vi "refocusProgram.vi"(8 "error in (no error)":errorcluster) -> ()   [LabVIEW 2022 SP3]
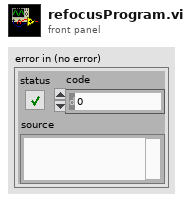
[diagram p1: front panel]
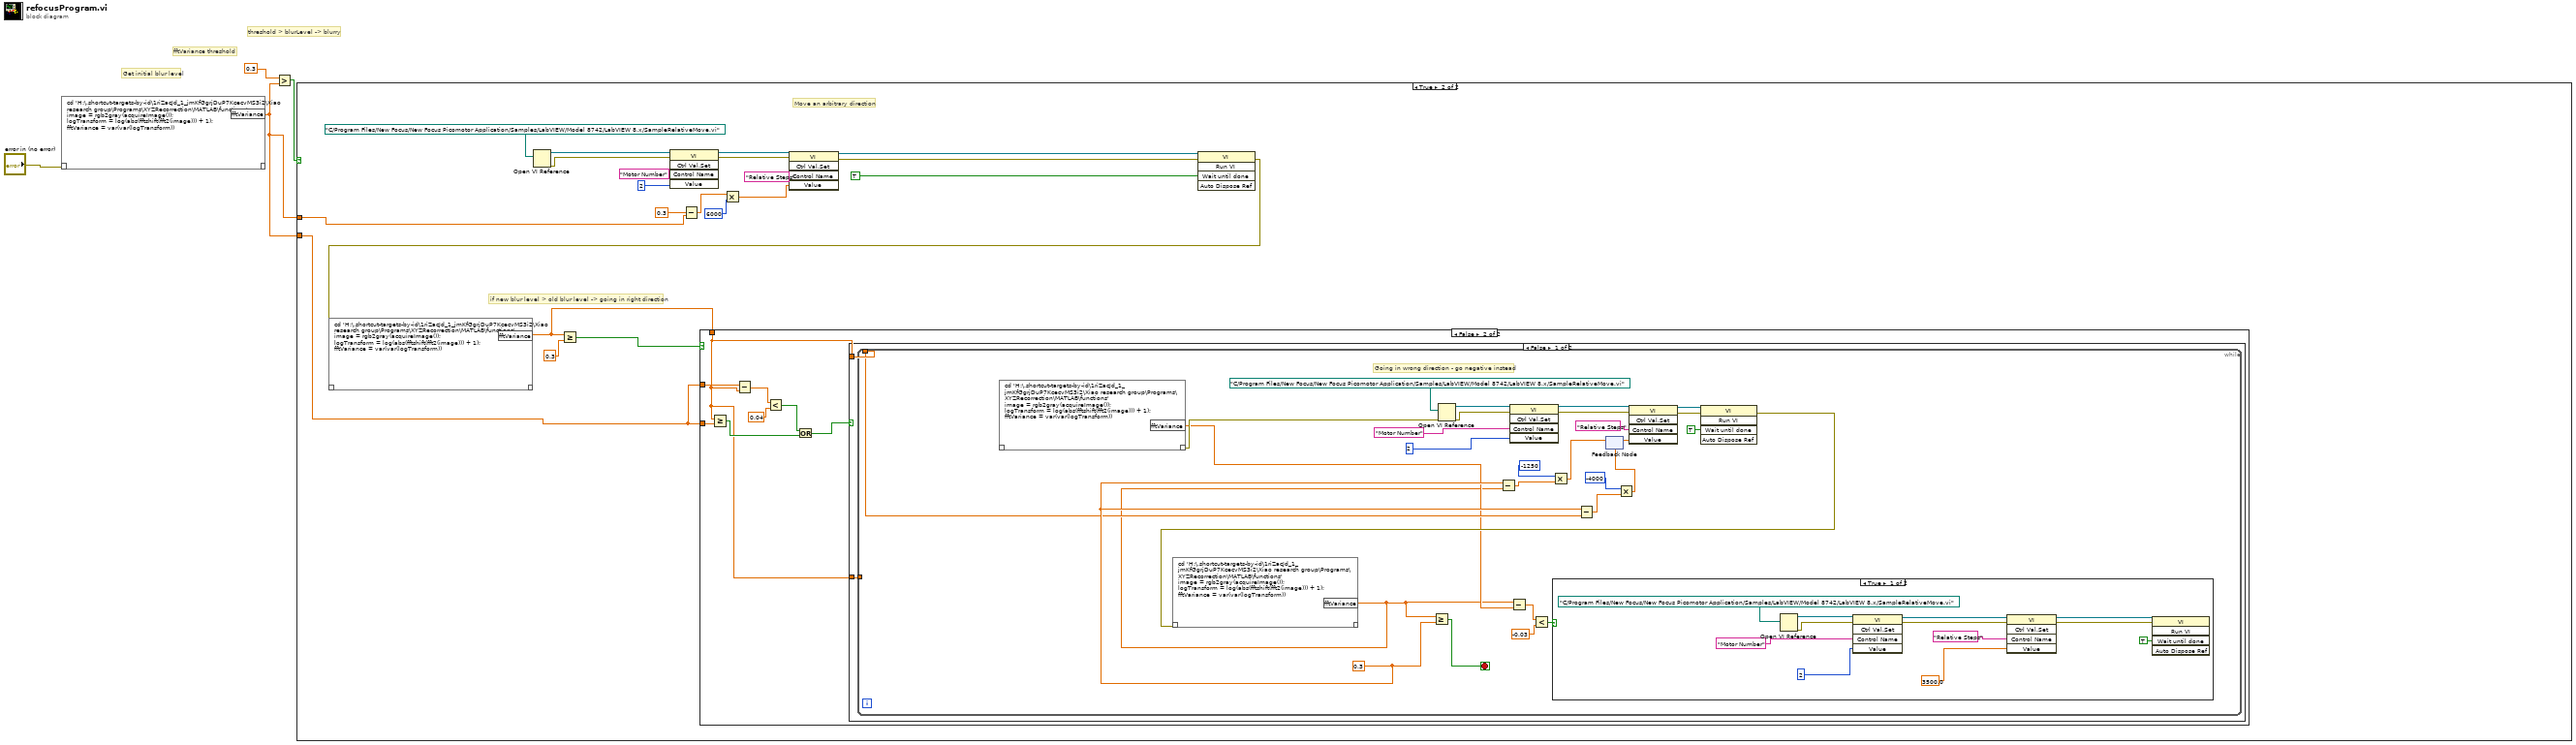
[diagram p0: block diagram]
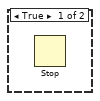
[diagram p3: hidden frame]
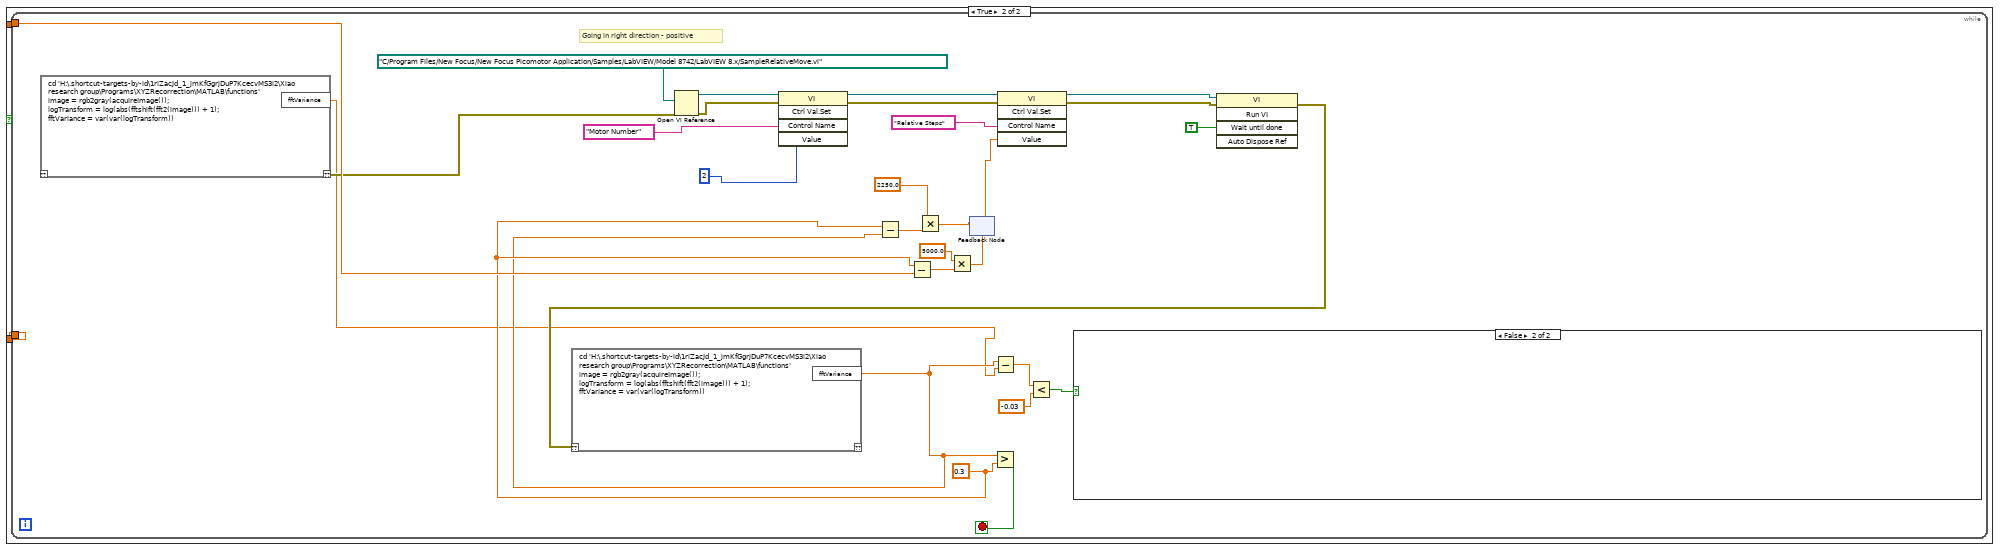
[diagram p5: hidden frame]
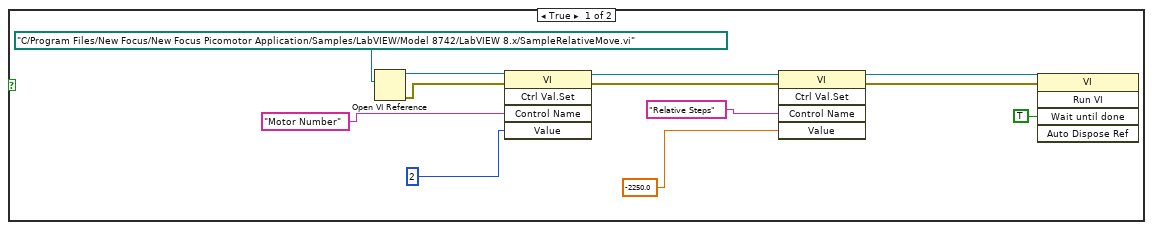
[diagram p6: hidden frame]
diagram:
  # "threshold > blurLevel -> blurry"
  # "fftVariance threshold"
  # "Get initial blur level"
  n1 = script code="cd 'H:\\.shortcut-targets-by-id\\1riZacJd_1_jmKfGgrjDuP7KcecvMS3i2\\Xiao research group\\Programs\\XYZRecorrection\\MATLAB\\functions'\nimage = rgb2gray(acquireImage());\nlogTransform = log(abs(fftshift(fft2(image))) + 1);\nfftVariance = var(var(logTransform))"("??"="error in (no error)") -> ("fftVariance"=w2:dbl)  [unwired: 1 out]
  n2 = Greater?(x=0.3, y=w2) -> (0:w4:bool)
  n3 = case shown="True" w4 {
    tunnel: w2 -> [_ w5]
    tunnel: w2 -> [_ w10]
    frame False {
      # "If the blurlevel is greater than the threshold value then the image is not blurry so continue with the program"
    }
    frame True {
      # "if new blur level > old blur level -> going in right direction"
      # "Move an arbitrary direction"
      n4 = Open VI Reference(vi path=path "C:/Program Files/New Focus/New Focus Picomotor Application/Samples/LabVIEW/Model 8742/LabVIEW 8.x/SampleRelativeMove.vi") -> (vi reference=w24:refnum<vi>, error out=w23:errorcluster)  [unwired: 5 in]
      n5 = invoke class="VI" method="Ctrl Val.Set"(reference=w24, error in=w23, "Control Name"="Motor Number", "Value"=2) -> (reference out=w21:refnum<vi>, error out=w20:errorcluster)  [unwired: 1 in, 3 out]
      n6 = Subtract(x=0.3, y=w10) -> (x-y=w9:dbl)
      n7 = Multiply(x=w9, y=6000) -> (x*y=w12:dbl)
      n8 = invoke class="VI" method="Ctrl Val.Set"(reference=w21, error in=w20, "Control Name"="Relative Steps", "Value"=w12) -> (reference out=w17:refnum<vi>, error out=w16:errorcluster)  [unwired: 1 in, 3 out]
      n9 = invoke class="VI" method="Run VI"(reference=w17, error in=w16, "Wait until done"=TRUE ("Wait Until Done")) -> (error out=w15:errorcluster)  [unwired: 2 in, 4 out]
      n10 = script code="cd 'H:\\.shortcut-targets-by-id\\1riZacJd_1_jmKfGgrjDuP7KcecvMS3i2\\Xiao research group\\Programs\\XYZRecorrection\\MATLAB\\functions'\nimage = rgb2gray(acquireImage());\nlogTransform = log(abs(fftshift(fft2(image))) + 1);\nfftVariance = var(var(logTransform))"("??"=w15) -> ("fftVariance"=w6:dbl)  [unwired: 1 out]
      n11 = Greater Or Equal?(x=w6, y=0.3) -> (x >= y?=w7:bool)
      n12 = case shown="False" w7 {
        tunnel: w5 -> [_ w33]
        tunnel: w6 -> [_ w26]
        tunnel: w5 -> [_ w29]
        frame True {
          n13 = Stop() -> ()  [unwired: 1 in]
        }
        frame False {
          n14 = Greater Or Equal?(x=w26, y=w33) -> (x >= y?=w32:bool)
          n15 = Subtract(x=w29, y=w26) -> (x-y=w28:dbl)
          n16 = Less?(x=w28, y=0.04) -> (x < y?=w27:bool)
          n17 = Or(x=w27, y=w32) -> (x .or. y?=w31:bool)
          n18 = case shown="False" w31 {
            tunnel: w26 -> [w35 w77]
            tunnel: w26 -> [w34 w76]
            frame False {
              n19 = while {
                tunnel: w35 -> [w43]
                tunnel: w34 -> [_]
                stop <- w52 stop-if-true
                w44 = 0.3
                # "Going in wrong direction - go negative instead"
                n20 = script code="cd 'H:\\.shortcut-targets-by-id\\1riZacJd_1_jmKfGgrjDuP7KcecvMS3i2\\Xiao research group\\Programs\\XYZRecorrection\\MATLAB\\functions'\nimage = rgb2gray(acquireImage());\nlogTransform = log(abs(fftshift(fft2(image))) + 1);\nfftVariance = var(var(logTransform))"() -> ("??"=w39:errorcluster, "fftVariance"=w38:dbl)  [unwired: 1 in]
                n21 = Open VI Reference(vi path=path "C:/Program Files/New Focus/New Focus Picomotor Application/Samples/LabVIEW/Model 8742/LabVIEW 8.x/SampleRelativeMove.vi", error in (no error)=w39) -> (vi reference=w62:refnum<vi>, error out=w61:errorcluster)  [unwired: 4 in]
                n22 = invoke class="VI" method="Ctrl Val.Set"(reference=w62, error in=w61, "Control Name"="Motor Number", "Value"=2) -> (reference out=w59:refnum<vi>, error out=w58:errorcluster)  [unwired: 1 in, 3 out]
                n23 = Subtract(x=w44, y=w43) -> (x-y=w46:dbl)
                n24 = Multiply(x=-4000, y=w46) -> (x*y=w42:dbl)
                n25 = feedback #1(w42) -> (w47:dbl)
                n26 = invoke class="VI" method="Ctrl Val.Set"(reference=w59, error in=w58, "Control Name"="Relative Steps", "Value"=w47) -> (reference out=w55:refnum<vi>, error out=w54:errorcluster)  [unwired: 1 in, 3 out]
                n27 = invoke class="VI" method="Run VI"(reference=w55, error in=w54, "Wait until done"=TRUE ("Wait Until Done")) -> (error out=w53:errorcluster)  [unwired: 2 in, 4 out]
                n28 = script code="cd 'H:\\.shortcut-targets-by-id\\1riZacJd_1_jmKfGgrjDuP7KcecvMS3i2\\Xiao research group\\Programs\\XYZRecorrection\\MATLAB\\functions'\nimage = rgb2gray(acquireImage());\nlogTransform = log(abs(fftshift(fft2(image))) + 1);\nfftVariance = var(var(logTransform))"("??"=w53) -> ("fftVariance"=w37:dbl)  [unwired: 1 out]
                n29 = Greater Or Equal?(x=w37, y=w44) -> (x >= y?=w52:bool)
                n30 = Subtract(x=w44, y=w37) -> (x-y=w50:dbl)
                n31 = Subtract(x=w37, y=w38) -> (x-y=w41:dbl)
                n32 = Less?(x=w41, y=-0.03) -> (x < y?=w36:bool)
                n33 = Multiply(x=-1250, y=w50) -> (x*y=w48:dbl)
                n34 = case shown="True" w36 {
                  frame True {
                    n35 = Open VI Reference(vi path=path "C:/Program Files/New Focus/New Focus Picomotor Application/Samples/LabVIEW/Model 8742/LabVIEW 8.x/SampleRelativeMove.vi") -> (vi reference=w75:refnum<vi>, error out=w74:errorcluster)  [unwired: 5 in]
                    n36 = invoke class="VI" method="Ctrl Val.Set"(reference=w75, error in=w74, "Control Name"="Motor Number", "Value"=2) -> (reference out=w73:refnum<vi>, error out=w72:errorcluster)  [unwired: 1 in, 3 out]
                    n37 = invoke class="VI" method="Ctrl Val.Set"(reference=w73, error in=w72, "Control Name"="Relative Steps", "Value"=3500.0 ("x")) -> (reference out=w71:refnum<vi>, error out=w70:errorcluster)  [unwired: 1 in, 3 out]
                    n38 = invoke class="VI" method="Run VI"(reference=w71, error in=w70, "Wait until done"=TRUE ("Wait Until Done")) -> ()  [unwired: 2 in, 5 out]
                  }
                  frame False {
                  }
                }
                n39 = feedback-in #1(w48) -> ()
              }
            }
            frame True {
              n40 = while {
                tunnel: w77 -> [w85]
                tunnel: w76 -> [_]
                stop <- w95 stop-if-true
                w84 = 0.3
                # "Going in right direction - positive"
                n41 = script code="cd 'H:\\.shortcut-targets-by-id\\1riZacJd_1_jmKfGgrjDuP7KcecvMS3i2\\Xiao research group\\Programs\\XYZRecorrection\\MATLAB\\functions'\nimage = rgb2gray(acquireImage());\nlogTransform = log(abs(fftshift(fft2(image))) + 1);\nfftVariance = var(var(logTransform))"() -> ("??"=w83:errorcluster, "fftVariance"=w79:dbl)  [unwired: 1 in]
                n42 = Open VI Reference(vi path=path "C:/Program Files/New Focus/New Focus Picomotor Application/Samples/LabVIEW/Model 8742/LabVIEW 8.x/SampleRelativeMove.vi", error in (no error)=w83) -> (vi reference=w104:refnum<vi>, error out=w103:errorcluster)  [unwired: 4 in]
                n43 = invoke class="VI" method="Ctrl Val.Set"(reference=w104, error in=w103, "Control Name"="Motor Number", "Value"=2) -> (reference out=w101:refnum<vi>, error out=w100:errorcluster)  [unwired: 1 in, 3 out]
                n44 = Subtract(x=w84, y=w85) -> (x-y=w88:dbl)
                n45 = Multiply(x=5000.0, y=w88) -> (x*y=w87:dbl)
                n46 = feedback #2(w87) -> (w89:dbl)
                n47 = invoke class="VI" method="Ctrl Val.Set"(reference=w101, error in=w100, "Control Name"="Relative Steps", "Value"=w89) -> (reference out=w97:refnum<vi>, error out=w96:errorcluster)  [unwired: 1 in, 3 out]
                n48 = invoke class="VI" method="Run VI"(reference=w97, error in=w96, "Wait until done"=TRUE ("Wait Until Done")) -> (error out=w94:errorcluster)  [unwired: 2 in, 4 out]
                n49 = script code="cd 'H:\\.shortcut-targets-by-id\\1riZacJd_1_jmKfGgrjDuP7KcecvMS3i2\\Xiao research group\\Programs\\XYZRecorrection\\MATLAB\\functions'\nimage = rgb2gray(acquireImage());\nlogTransform = log(abs(fftshift(fft2(image))) + 1);\nfftVariance = var(var(logTransform))"("??"=w94) -> ("fftVariance"=w80:dbl)  [unwired: 1 out]
                n50 = Subtract(x=w84, y=w80) -> (x-y=w92:dbl)
                n51 = Multiply(x=2250.0, y=w92) -> (x*y=w90:dbl)
                n52 = feedback-in #2(w90) -> ()
                n53 = Greater?(x=w80, y=w84) -> (0:w95:bool)
                n54 = Subtract(x=w80, y=w79) -> (x-y=w78:dbl)
                n55 = Less?(x=w78, y=-0.03) -> (x < y?=w81:bool)
                n56 = case shown="False" w81 {
                  frame True {
                    n57 = Open VI Reference(vi path=path "C:/Program Files/New Focus/New Focus Picomotor Application/Samples/LabVIEW/Model 8742/LabVIEW 8.x/SampleRelativeMove.vi") -> (vi reference=w117:refnum<vi>, error out=w116:errorcluster)  [unwired: 5 in]
                    n58 = invoke class="VI" method="Ctrl Val.Set"(reference=w117, error in=w116, "Control Name"="Motor Number", "Value"=2) -> (reference out=w115:refnum<vi>, error out=w114:errorcluster)  [unwired: 1 in, 3 out]
                    n59 = invoke class="VI" method="Ctrl Val.Set"(reference=w115, error in=w114, "Control Name"="Relative Steps", "Value"=-2250.0 ("x")) -> (reference out=w113:refnum<vi>, error out=w112:errorcluster)  [unwired: 1 in, 3 out]
                    n60 = invoke class="VI" method="Run VI"(reference=w113, error in=w112, "Wait until done"=TRUE ("Wait Until Done")) -> ()  [unwired: 2 in, 5 out]
                  }
                  frame False {
                  }
                }
              }
            }
          }
        }
      }
    }
  }
